vi "Agilent DMM Read Resolution.vi"(7 "Measurement Type":T3, 8 "error in (no error)":errorcluster, 10 "Range":T1, 11 "VISA Resource Name":refnum<visa-resource-name>) -> (0 "error out":errorcluster, 2 "Resolution":T2, 3 "dup VISA Resource Name":refnum<visa-resource-name>)   [LabVIEW 2011]
doc: "This VI for the HP 8753 is used to read the sweep type.\n\n0 LINEAR FREQ\n1 LOG FREQ\n2 LIST FREQ\n3 CW TIME\n4 POWER SWEEP"
uses:
  TypeDefs/Agilent DMM Measurement Type.ctl
  TypeDefs/Agilent DMM Resolution.ctl
  TypeDefs/Agilent DMM Range.ctl
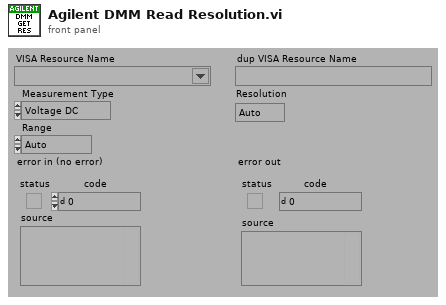
[diagram p1: front panel]
types:
  T1 = typedef "Agilent DMM Range.ctl" = enum16{"Auto", "Min", "Max", "0.01", "0.1", "1", "3", "10", "100", "1,000", "10,000", "100,000", "1,000,000", "10,000,000", "100,000,000"}
  T2 = typedef "Agilent DMM Resolution.ctl" = enum16{"Auto", "Min", "Max", "4 1/2", "5 1/2", "6 1/2"}
  T3 = typedef "Agilent DMM Measurement Type.ctl" = enum16{"Voltage DC", "Voltage DC Ratio", "Voltage AC", "Current DC", "Current AC", "Resistance", "Fresistance", "Frequency", "Period", "Continuity", "Diode"}
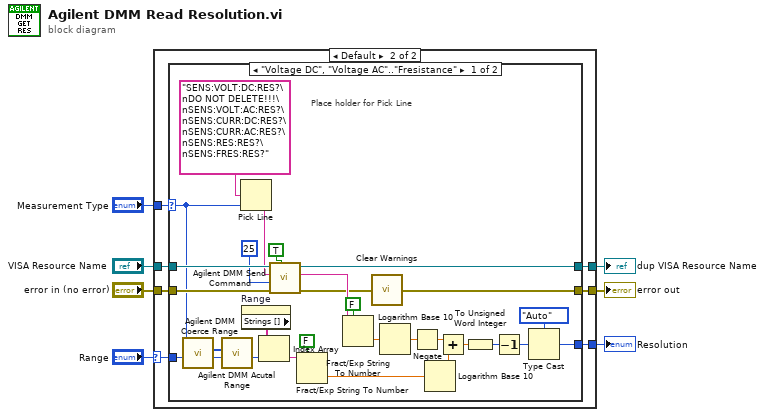
[diagram p0: block diagram]
diagram:
  n1 = case shown="Default" "Range" {
    selector: "Range" -> [_ w10]
    tunnel: "error in (no error)" -> [w9 w16]
    tunnel: [w9 w15] -> w6
    tunnel: "VISA Resource Name" -> [w8 w14]
    tunnel: [w8 w13] -> w4
    tunnel: "Measurement Type" -> [_ w12]
    tunnel: [_ w11] -> w2
    frame "Auto" {
      # "The Resolution is Auto when the Range is Auto."
    }
    frame Default {
      n2 = case shown="\"Voltage DC\", \"Voltage AC\"..\"Fresistance\"" w12 {
        selector: w12 -> [w32 _]
        tunnel: w16 -> [w42 w47]
        tunnel: [w23 w47] -> w15
        tunnel: w14 -> [w43 w46]
        tunnel: [w20 w46] -> w13
        tunnel: [w33 _] -> w11
        tunnel: w10 -> [w31 _]
        frame "Voltage DC", "Voltage AC".."Fresistance" {
          # "Place holder for Pick Line"
          n3 = call "Agilent DMM Coerce Range.vi"("Range"=w31, "Measurement Type"=w32) -> ("Coerced Range"=w26:T1, "Available Ranges"=w24:T1[])  [unwired: 8 out]
          n4 = call "Agilent DMM Acutal Range.vi"("Coerced Range"=w26, "Available Ranges"=w24) -> ("Acutal Range"=w25:T1)  [unwired: 9 out]
          n5 = Pick Line(multi-line string="SENS:VOLT:DC:RES?\nDO NOT DELETE!!!\nSENS:VOLT:AC:RES?\nSENS:CURR:DC:RES?\nSENS:CURR:AC:RES?\nSENS:RES:RES?\nSENS:FRES:RES?" ("write buffer"), line index=w32) -> (output string=w22:string)  [unwired: 1 out]
          n6 = property on="Range" class="Enum (strict)"() -> ("Strings []"=w30:string[])  [unwired: 2 in, 2 out]
          n7 = Index Array(array=w30, index=w25) -> (element=w29:string)
          n8 = call "Agilent DMM Send Command.vi"("Read? (F)"=TRUE, "error in (no error)"=w42, "Byte Count"=u32 25, "Command"=w22, "VISA Resource Name"=w43) -> ("error out"=w19:errorcluster, "Data Read"=w21:string, "dup VISA Resource Name"=w20:refnum<visa-resource-name>)  [unwired: 4 out]
          n9 = Fract/Exp String To Number(use system decimal point (T)=FALSE, string=w29) -> (number=w27:dbl)  [unwired: 3 out]
          n10 = Fract/Exp String To Number(use system decimal point (T)=FALSE, string=w21) -> (number=w38:dbl)  [unwired: 3 out]
          n11 = call "Clear Warnings.vi"("error in (no error)"=w19) -> ("error out"=w23:errorcluster)
          n12 = Logarithm Base 10(1:w38) -> (0:w39:dbl)
          n13 = Negate(x=w39) -> (-x=w40:dbl)
          n14 = Logarithm Base 10(1:w27) -> (0:w41:dbl)
          n15 = Add(x=w40, y=w41) -> (x+y=w37:dbl)
          n16 = To Unsigned Word Integer(number=w37) -> (unsigned 16bit integer=w36:u16)
          n17 = Decrement(x=w36) -> (x-1=w35:u16)
          n18 = Type Cast(type=Agilent_DMM_Resolution."Auto" ("Resolution"), x=w35) -> (*(type *) &x=w33:T2)
        }
        frame Default {
          # "The Resolution can not be read for:\n\nVoltage DC Ratio,\nFrequency,\nPeriod,\nContinuity, or\nDiode."
        }
      }
    }
  }
  "dup VISA Resource Name" <- w4
  "error out" <- w6
  "Resolution" <- w2
